vi "IV setcellon.vi"(8 "error in (no error)":errorcluster, 11 "cellon":i32) -> (0 "error out":errorcluster, 2 "return type":i32, 3 "cellon out":i32)   [LabVIEW 2020, in "IVIUM_remdriver.lvlib"]
uses:
  Labview/IVIUM/IVIUM_remdriver.lvlib
  Labview/IVIUM/IVIUM_remdriver.dll
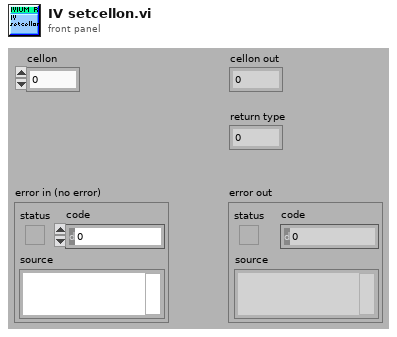
[diagram p1: front panel]
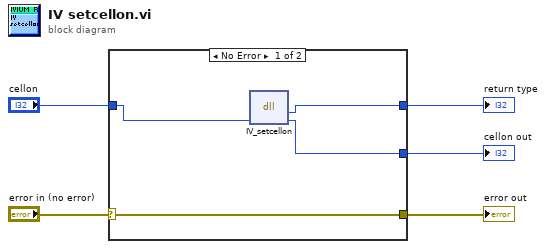
[diagram p0: block diagram]
diagram:
  n1 = case shown="No Error" "error in (no error)" {
    selector: "error in (no error)" -> [w9 w11]
    tunnel: [w9 w11] -> w4
    tunnel: [w8 _] -> w3
    tunnel: "cellon" -> [w7 w10]
    tunnel: [w6 w10] -> w1
    frame No Error {
      n2 = dll-call lib="C:/SEC Software V4.0/Labview/IVIUM/IVIUM_remdriver.*" fn="IV_setcellon"("cellon"=w7) -> (w8:i32, "cellon"=w6:i32)  [unwired: 3 in, 2 out]
    }
    frame Error {
    }
  }
  "return type" <- w3
  "cellon out" <- w1
  "error out" <- w4
